vi "Test - Draw Filled Triangle.vi"() -> ()   [LabVIEW 2022 SP3, in "Raster.lvlib"]
uses:
  Raster.lvlib
  Utility/Utility.lvlib
  Rectangle Dimensions.ctl
  5ea285c7-be76-47ab-bb95-511c6a9aac96.vi
  d84cddbd-8e40-43c7-a758-6e8d8fd6f2c6.vi
  Point 2D.ctl
panel:
  in  "Point 3":T1={"x"=0, "y"=200}
  in  "Point 2":T1={"x"=100, "y"=100}
  in  "Point 1":T1
  out "Time [s]":dbl format="%.3p"
  out "new picture":picture
  # "(0,0)"
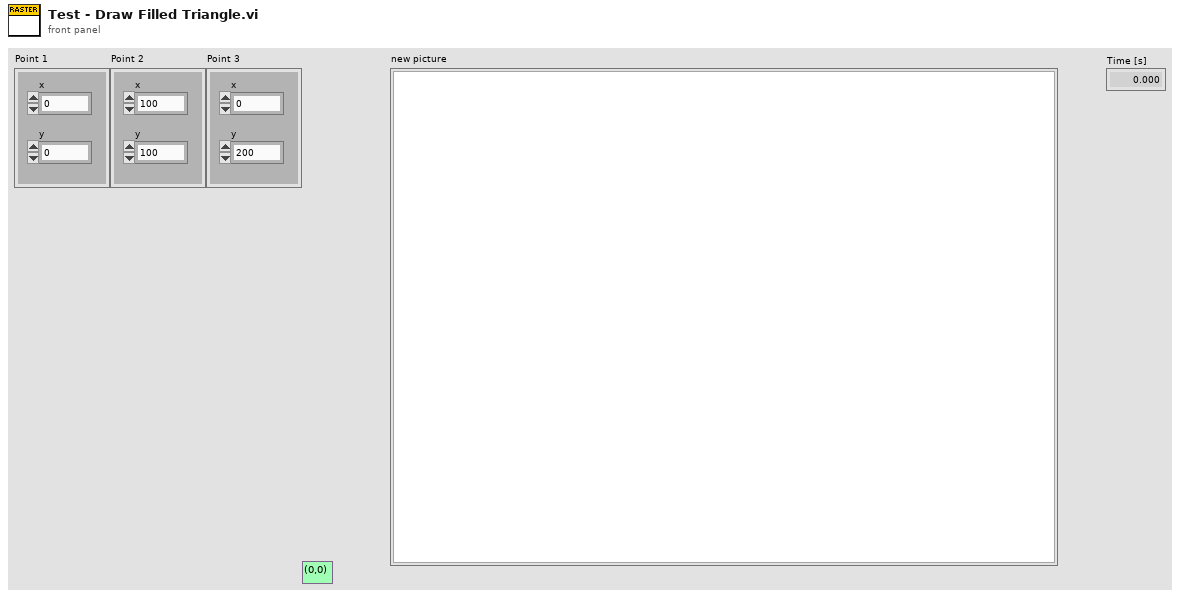
[diagram p1: front panel]
types:
  T1 = typedef "Raster.lvlib/Point 2D.ctl" = cluster{"x":i32, "y":i32}
  T2 = typedef "Raster.lvlib/Rectangle Dimensions.ctl" = cluster{"Width":u32, "Height":u32}
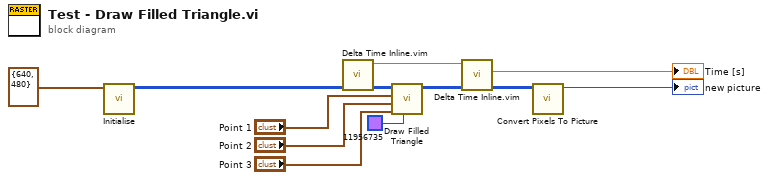
[diagram p0: block diagram]
diagram:
  n1 = call "Initialise.vi"("Screen Dimensions"=T2 {"Width"=640, "Height"=480}) -> ("Pixel Data out"=w6:u32[][])  [unwired: 10 in]
  n2 = call "Delta Time Inline.vim"("value in"=w6) -> ("value out"=w5:u32[][], "Relative Seconds out [s]"=w1:dbl)  [unwired: 8 in, 1 out]
  n3 = call "Draw Filled Triangle.vi"("Fill Colour"=u32 11956735 ("Line Colour"), "Point 3"="Point 3", "Point 2"="Point 2", "Point 1"="Point 1", "Pixel Data in"=w5) -> ("Pixel Data out"=w4:u32[][])  [unwired: 6 in]
  n4 = call "Delta Time Inline.vim"("value in"=w4, "Relative Seconds in [s]"=w1) -> ("value out"=w3:u32[][], "Delta Time [s]"=→"Time [s]":dbl)  [unwired: 7 in, 1 out]
  n5 = call "Convert Pixels To Picture.vi"("Pixel Data in"=w3) -> ("2D Picture"=→"new picture":picture)  [unwired: 9 in, 1 out]
